vi "qHIS.vi"(0 "System no.":i32=1 min=1 max=4 step=1, 2 "DeviceID":i32=1, 3 "Property":i32=1, 4 "Query selection":T1(ring), 5 "error in":errorcluster, 6 "ItemID":i32=1) -> (14 "HIS? Answer string":string, 19 "error out":errorcluster)   [LabVIEW 2026]
doc: "This VI returns a list of Human Interface Devices (HID) connected to the controller, their items, properties and values and queries error. See controller user manual for details. \n\nC-867:"
panel:
  # "This vi returns a list of Human Interface Devices (HID) connected to the controller, their \nitems, properties and values and queries error. See controller User Manual for details."
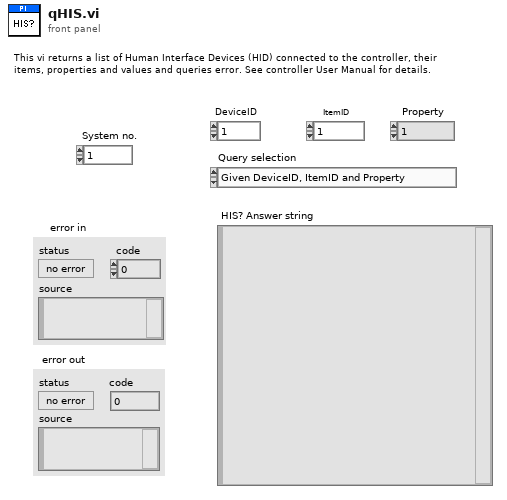
[diagram p1: front panel]
types:
  T1 = enum16{"Given DeviceID, ItemID and Property", "Given DeviceID and ItemID, all Properties", "Given DeviceID, all ItemIDs and Properties", "All DeviceIDs, ItemIDs and Properties"}
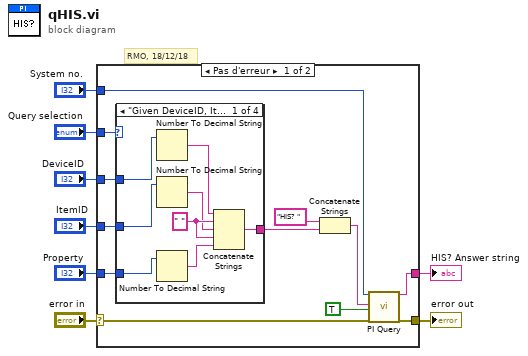
[diagram p0: block diagram]
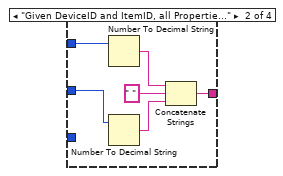
[diagram p2: hidden frame]
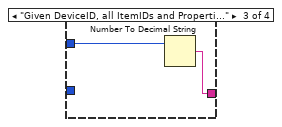
[diagram p3: hidden frame]
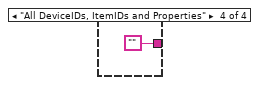
[diagram p4: hidden frame]
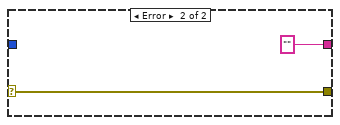
[diagram p5: hidden frame]
diagram:
  # "RMO, 18/12/18"
  n1 = case shown="Pas d'erreur" "error in" {
    selector: "error in" -> [w10 w38]
    tunnel: "System no." -> [w20 _]
    tunnel: [w9 w38] -> w7
    tunnel: [w11 "" ("String read")] -> w6
    tunnel: "Query selection" -> [w12 _]
    tunnel: "DeviceID" -> [w15 _]
    tunnel: "ItemID" -> [w14 _]
    tunnel: "Property" -> [w13 _]
    frame No Error {
      n2 = case shown="\"Given DeviceID, ItemID and Property\", Par défaut" w12 {
        tunnel: [w27 w31 w36 ""] -> w16
        tunnel: w15 -> [w28 w30 w35 _]
        tunnel: w14 -> [w26 w29 _ _]
        tunnel: w13 -> [w25 _ _ _]
        frame "Given DeviceID, ItemID and Property", Default {
          w24 = " " ("string")
          n3 = Number To Decimal String(number=w28) -> (decimal integer string=w23:string)  [unwired: 1 out]
          n4 = Number To Decimal String(number=w26) -> (decimal integer string=w22:string)  [unwired: 1 out]
          n5 = Number To Decimal String(number=w25) -> (decimal integer string=w21:string)  [unwired: 1 out]
          n6 = Concatenate Strings(w23, w24, w22, w24, w21) -> (w27:string)
        }
        frame "Given DeviceID and ItemID, all Properties" {
          n7 = Number To Decimal String(number=w30) -> (decimal integer string=w34:string)  [unwired: 1 out]
          n8 = Number To Decimal String(number=w29) -> (decimal integer string=w33:string)  [unwired: 1 out]
          n9 = Concatenate Strings(w34, " " ("string"), w33) -> (w31:string)
        }
        frame "Given DeviceID, all ItemIDs and Properties" {
          n10 = Number To Decimal String(number=w35) -> (decimal integer string=w36:string)  [unwired: 1 out]
        }
        frame "All DeviceIDs, ItemIDs and Properties" {
        }
      }
      n11 = Concatenate Strings("HIS? ", w16) -> (w17:string)
      n12 = call "PI Query.vi"("System no."=w20, "String to send"=w17, "Attach termination char.?"=TRUE ("Attach Linefeed?"), "error in"=w10) -> ("String read"=w11:string, "error out"=w9:errorcluster)  [unwired: 3 in, 11 out]
    }
    frame Error {
    }
  }
  "error out" <- w7
  "HIS? Answer string" <- w6
